vi "Get History Chart.vi"(10 "duration":dbl, 11 "Stock Name":string) -> (3 "new picture":picture)   [LabVIEW 2025, in "Full Featured MCP Server.lvlib"]
doc: "Returns a picture of a graph of the specified stock for the last time specified by duration."
uses:
  Full Featured MCP Server.lvlib
panel:
  out "Response":string
  out "Waveform Graph":dbl[](graph)
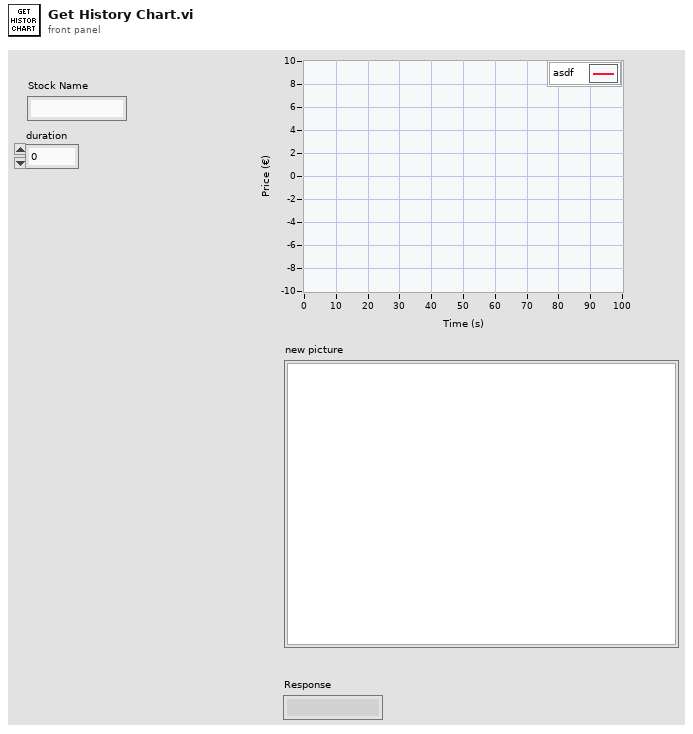
[diagram p1: front panel]
types:
  T1 = typedef "Full Featured MCP Server.lvlib/Server Data.ctl" = cluster{"Stocks Prices":dbl[][], "Owned Stocks":i32[], "Stock Names":string[], "Wallet":dbl, "Fluctuation":dbl, "Stock Trends":dbl[]}
  T2 = typedef "imagedata.ctl" = cluster{"image type":i32, "image depth":i32, "image":u8[], "mask":u8[], "colors":u32[], "Rectangle":cluster{"left":i16, "top":i16, "right":i16, "bottom":i16}}
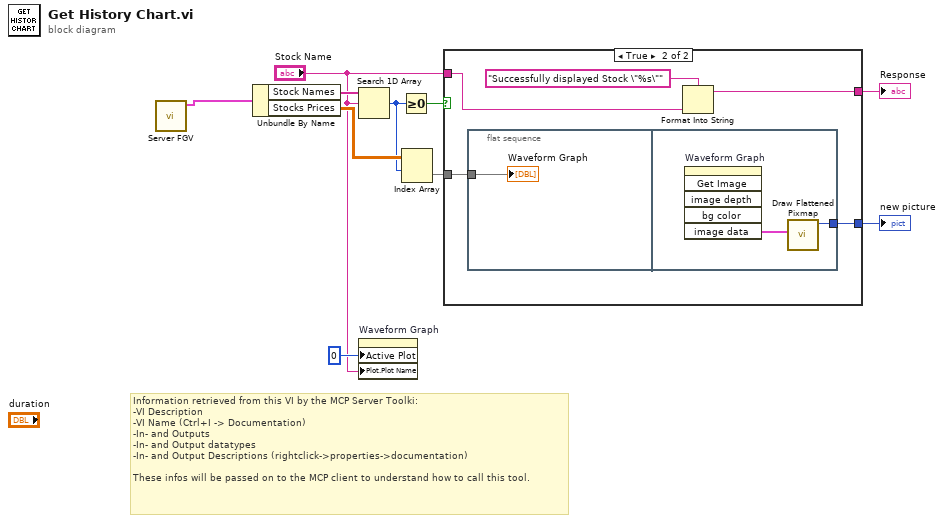
[diagram p0: block diagram]
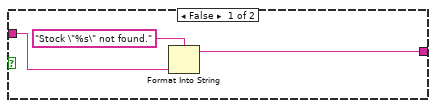
[diagram p2: hidden frame]
diagram:
  # "Information retrieved from this VI by the MCP Server Toolki:\n-VI Description\n-VI Name (Ctrl+I -> Documentation)\n-In- and Outputs\n-In- and Output datatypes\n-In- and Output Descriptions (rightclick->properties->documentation)\n\nThese infos will be passed on to the MCP client to understand how to call this tool."
  n1 = call "Server FGV.vi"() -> ("Full Features MCP Server Data"=w1:T1)  [unwired: 9 in, 2 out]
  n2 = Unbundle By Name(w1) -> ("Stock Names"=w10:string[], "Stocks Prices"=w9:dbl[][])
  n3 = Search 1D Array(1D array=w10, element="Stock Name") -> (index of element=w8:i32)  [unwired: 1 in]
  n4 = property on="Waveform Graph" class="WFGraph (strict)"("Active Plot"=u32 0, "Plot.Plot Name"="Stock Name") -> ()  [unwired: 2 in, 2 out]
  n5 = Greater Or Equal To 0?(x=w8) -> (x >= 0?=w4:bool)
  n6 = Index Array(array=w9, index (row)=w8) -> (element=w6:dbl[])  [unwired: 1 in]
  n7 = case shown="True" w4 {
    tunnel: w6 -> [_ w18]
    tunnel: [_ w17] -> w5
    tunnel: "Stock Name" -> [w12 w15]
    tunnel: [w11 w14] -> w2
    frame False {
      n8 = Format Into String(format string="Stock \"%s\" not found.", w12) -> (resulting string=w11:string)  [unwired: 2 in, 1 out]
    }
    frame True {
      n9 = flat-sequence {
        tunnel: w18 -> [w19]
        tunnel: [w20] -> w17
        frame #0 {
          "Waveform Graph" <- w19
        }
        frame #1 {
          n10 = invoke on="Waveform Graph" class="WFGraph (strict)" method="Get Image"() -> ("image data"=w21:T2)  [unwired: 6 in, 5 out]
          n11 = call <vilib>:"Draw Flattened Pixmap.vi"("image data"=w21) -> ("new picture"=w20:picture)  [unwired: 8 in]
        }
      }
      n12 = Format Into String(format string="Successfully displayed Stock \"%s\"", w15) -> (resulting string=w14:string)  [unwired: 2 in, 1 out]
    }
  }
  "Response" <- w2
  "new picture" <- w5
